vi "Buttons.vi"(8 "Joystick Name":string, 9 "Button Not Pressed Speed":dbl, 10 "Button Pressed Speed":dbl, 11 "Button Index":dbl) -> (3 "Numeric":dbl)   [LabVIEW 2019]
uses:
  <vilib>/Rock Robotics/WPI/Utilities/WPI_GetSetVariantRefNum.vi
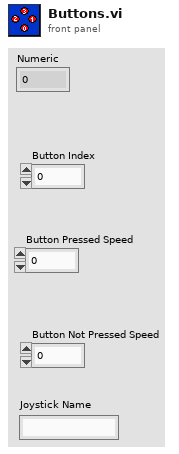
[diagram p1: front panel]
types:
  T1 = typedef "WPI_JoystickDevRef.ctl" = cluster{"Device":T2}
  T2 = typedef "WPI_JoystickDeviceEnum.ctl" = enum16{"USB 0", "USB 1", "USB 2", "USB 3", "USB 4", "USB 5"}
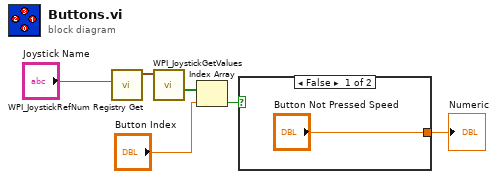
[diagram p0: block diagram]
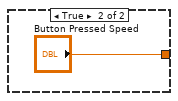
[diagram p2: hidden frame]
diagram:
  n1 = call <vilib>:"WPI_JoystickRefNum Registry Get.vi"("refnum name"="Joystick Name") -> ("JoystickDevRef"=w3:T1)  [unwired: 1 in, 9 out]
  n2 = call <vilib>:"WPI_JoystickGetValues.vi"("JoystickDevRef"=w3) -> ("Buttons"=w4:bool[])  [unwired: 6 in, 4 out]
  n3 = Index Array(array=w4, index="Button Index") -> (element=w6:bool)
  n4 = case shown="False" w6 {
    tunnel: ["Button Not Pressed Speed" "Button Pressed Speed"] -> w5
    frame False {
    }
    frame True {
    }
  }
  "Numeric" <- w5
